vi "Climb Encoder.vi"(10 "Reset":bool, 11 "Enum":enum16{"Start", "Run", "End"}(ring)) -> (3 "Distance":dbl)   [LabVIEW 2012]
uses:
  TypeDefs/Digital Module 1.ctl
  <vilib>/Rock Robotics/SystemInterfaces/Typedef/FPGA_TypedefDigitalModule.ctl
  <vilib>/Rock Robotics/SystemInterfaces/DIO/FPGA_DIOChannel.ctl
  <vilib>/Rock Robotics/WPI/Counter/WPI_CounterDigitalInputToDigitalSource.vi
panel:
  in  "Digital Module A":T1={"Module"=enum."Digital Module 1", "Base Limit Switch"=enum."DIO 1", "Top Limit Switch"=enum."DIO 2", "Dummy Limit Switch"=enum."DIO 3", "Compressor Switch"=enum."DIO 4", "Tachometer"=enum."DIO 5", "Encoder A"=enum."DIO 6", "Encoder B"=enum."DIO 7", "Unassigned"=enum."DIO 8", "Unassigned"=enum."DIO 9", "Unassigned"=enum."DIO 10", "Unassigned"=enum."DIO 11", "Unassigned"=enum."DIO 12", "Unassigned"=enum."DIO 13", "Unassigned"=enum."DIO 14"}
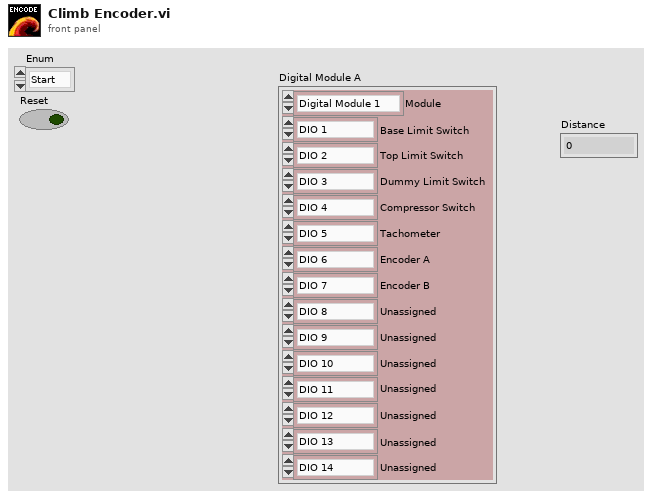
[diagram p1: front panel]
types:
  T1 = typedef "Digital Module 1.ctl" = cluster{"Module":T2, "Base Limit Switch":T3, "Top Limit Switch":T3, "Dummy Limit Switch":T3, "Compressor Switch":T3, "Tachometer":T3, "Encoder A":T3, "Encoder B":T3, "Unassigned":T3, "Unassigned":T3, "Unassigned":T3, "Unassigned":T3, "Unassigned":T3, "Unassigned":T3, "Unassigned":T3}
  T2 = typedef "FPGA_TypedefDigitalModule.ctl" = enum16{"Digital Module 1", "Digital Module 2"}
  T3 = typedef "FPGA_DIOChannel.ctl" = enum8{"DIO 1", "DIO 2", "DIO 3", "DIO 4", "DIO 5", "DIO 6", "DIO 7", "DIO 8", "DIO 9", "DIO 10", "DIO 11", "DIO 12", "DIO 13", "DIO 14", "Invalid"}
  T4 = typedef "WPI_DigitalInputDevRef.ctl" = cluster{"DevStatus":errorcluster, "DIO Channel":T3, "Digital Module":T2}
  T5 = typedef "FPGA_CounterEncoderSourceConvertionLVSourceType.ctl" = cluster{"DevStatus":errorcluster, "AnalogTriggerMode?":bool, "DigitalMode":cluster{"Digital Module":T2, "DIO Channel":T6}, "AnalogTriggerMode":cluster{"AnalogTriggerIndex":T7, "OutputType":T8}}
  T6 = typedef "FPGA_DIODigitalSourceChannel.ctl" = enum8{"DIO 1", "DIO 2", "DIO 3", "DIO 4", "DIO 5", "DIO 6", "DIO 7", "DIO 8", "DIO 9", "DIO 10", "DIO 11", "DIO 12", "DIO 13", "DIO 14", "Disabled"}
  T7 = typedef "FPGA_AnalogTriggerIndex.ctl" = enum8{"Trig 0", "Trig 1", "Trig 2", "Trig 3", "Trig 4", "Trig 5", "Trig 6", "Trig 7", "Invalid"}
  T8 = typedef "FPGA_AnalogTriggerOutType.ctl" = enum16{"InWindow", "TriggerState", "Rising", "Falling"}
  T9 = typedef "WPI_EncoderDevRef.ctl" = cluster{"DevStatus":errorcluster, "EncoderIndex":T10, "CounterIndex":T11, "DistancePerCount":dbl, "Decoding Type":T12}
  T10 = typedef "FPGA_EncoderIdx.ctl" = enum8{"Enc 0", "Enc 1", "Enc 2", "Enc 3", "Invalid"}
  T11 = typedef "FPGA_CounterCtrSystemIndex.ctl" = enum8{"Ctr 0", "Ctr 1", "Ctr 2", "Ctr 3", "Ctr 4", "Ctr 5", "Ctr 6", "Ctr 7", "Invalid"}
  T12 = typedef "WPI_EncoderType.ctl" = enum16{"1x", "2x", "4x"}
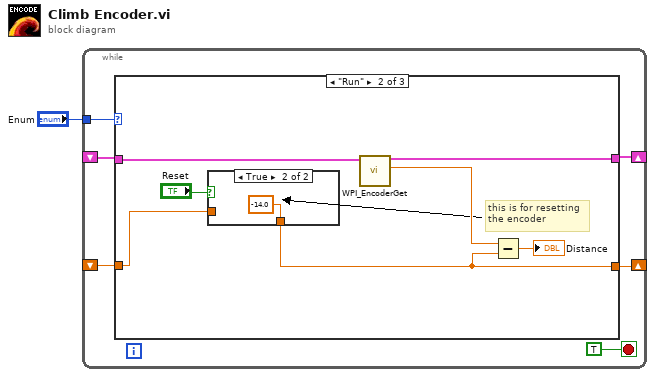
[diagram p0: block diagram]
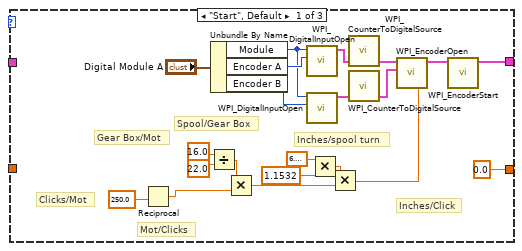
[diagram p2: hidden frame]
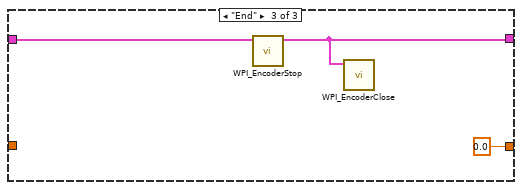
[diagram p4: hidden frame]
diagram:
  n1 = while {
    tunnel: "Enum" -> [w7]
    shift-right: [w6] -> _
    shift-left: _ -> [w5]
    shift-right: [w3] -> _
    shift-left: _ -> [w2]
    stop <- TRUE stop-if-true
    n2 = case shown="\"Run\"" w7 {
      tunnel: [w19 w35 w39] -> w6
      tunnel: w5 -> [_ w29 w40]
      tunnel: [0.0 ("Distance") w31 0.0 ("Distance")] -> w3
      tunnel: w2 -> [_ w33 _]
      frame "Start", Default {
        # "Inches/Click"
        # "Mot/Clicks"
        # "Gear Box/Mot"
        # "Inches/spool turn"
        # "Spool/Gear Box"
        # "Clicks/Mot"
        n3 = Reciprocal(x=250.0 ("y")) -> (1/x=w12:dbl)
        n4 = Divide(x=16.0, y=22.0) -> (x/y=w15:dbl)
        n5 = Unbundle By Name("Digital Module A") -> ("Module"=w24:T2, "Encoder A"=w25:T3, "Encoder B"=w23:T3)
        n6 = Multiply(x=w15, y=w12) -> (x*y=w13:dbl)
        n7 = call <vilib>:"WPI_DigitalInputOpen.vi"("DIO Channel"=w25, "Digital Module (Module 1)"=w24) -> ("DigitalInputDevRef"=w28:T4)  [unwired: 8 in, 1 out]
        n8 = call <vilib>:"WPI_DigitalInputOpen.vi"("DIO Channel"=w23, "Digital Module (Module 1)"=w24) -> ("DigitalInputDevRef"=w22:T4)  [unwired: 8 in, 1 out]
        n9 = Multiply(x=6.283185307179586, y=1.1532) -> (x*y=w10:dbl)
        n10 = Multiply(x=w10, y=w13) -> (x*y=w14:dbl)
        n11 = call-poly <vilib>:"WPI_CounterToDigitalSource.vi"("DigitalInputDevRef"=w28) -> ("Digital Source"=w27:T5)  [unwired: 6 in]
        n12 = call-poly <vilib>:"WPI_CounterToDigitalSource.vi"("DigitalInputDevRef"=w22) -> ("Digital Source"=w21:T5)  [unwired: 6 in]
        n13 = call <vilib>:"WPI_EncoderOpen.vi"("DistancePerCount"=w14, "BSource"=w21, "ASource"=w27) -> ("EncoderDevRef"=w20:T9)  [unwired: 7 in, 1 out]
        n14 = call <vilib>:"WPI_EncoderStart.vi"("EncoderDevRef"=w20) -> ("EncoderDevRef"=w19:T9)  [unwired: 9 in, 1 out]
      }
      frame "Run" {
        # "this is for resetting \nthe encoder"
        n15 = case shown="True" "Reset" {
          tunnel: [w36 -14.0 ("Distance")] -> w31
          tunnel: w33 -> [w36 _]
          frame False {
          }
          frame True {
          }
        }
        n16 = call <vilib>:"WPI_EncoderGet.vi"("EncoderDevRef"=w29) -> ("Distance"=w32:dbl, "EncoderDevRef"=w35:T9)  [unwired: 5 in, 4 out]
        n17 = Subtract(x=w32, y=w31) -> (x-y=→"Distance":dbl)
      }
      frame "End" {
        n18 = call <vilib>:"WPI_EncoderStop.vi"("EncoderDevRef"=w40) -> ("EncoderDevRef"=w39:T9)  [unwired: 9 in, 1 out]
        n19 = call <vilib>:"WPI_EncoderClose.vi"("EncoderDevRef"=w39) -> ()  [unwired: 10 in, 1 out]
      }
    }
  }
